vi "hEXLIFY.vi"(8 "error in (no error)":errorcluster, 11 "H Array":u32[](array[numeric])) -> (0 "error out":errorcluster, 3 "String":string)   [LabVIEW 2012, in "SHA256.lvlib"]
doc: "Convert an array of U32 words into a string of hex digits"
uses:
  SHA256.lvlib
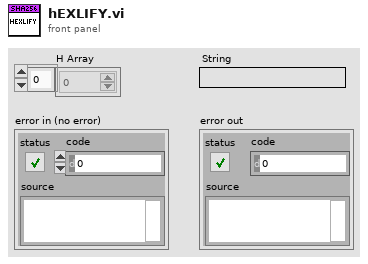
[diagram p1: front panel]
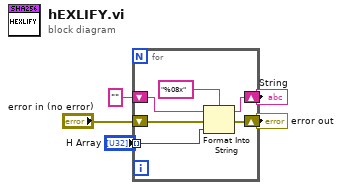
[diagram p0: block diagram]
diagram:
  n1 = for {
    tunnel: "H Array" -> [w11] mode=indexing
    shift-right: [w10] -> w3
    shift-left: "" -> [w9]
    shift-right: [w7] -> w4
    shift-left: "error in (no error)" -> [w6]
    n2 = Format Into String(format string="%08x", initial string=w9, error in=w6, w11) -> (resulting string=w10:string, error out=w7:errorcluster)
  }
  "error out" <- w4
  "String" <- w3
